vi "vi_tree.vi"   [LabVIEW 2010, in "zeromq.lvlib"]
uses:
  zeromq.lvlib
  poll_event_data.ctl
  zmq_context.lvclass
  zmq_socket.lvclass
  zmq_getsocketopt_int.vi
  zmq_poll_scalar.vi
panel:
  # "See back-panel for VI tree"
types:
  T1 = typedef "zeromq.lvlib/poll_event_data.ctl" = cluster{"identity":string, "data":string[]}
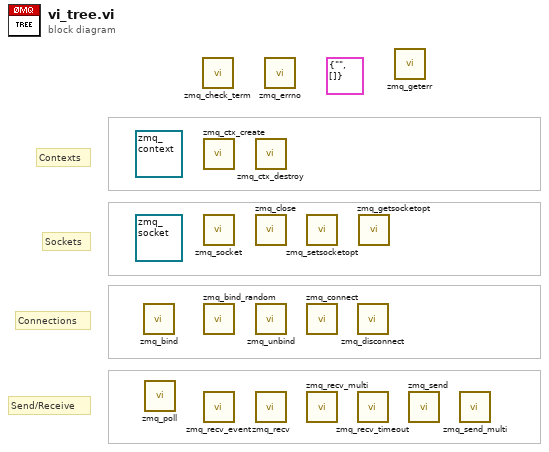
[diagram p0: block diagram]
diagram:
  (unwired) refnum<class "zmq_socket.lvclass"> refnum ("zeromq.lvlib:ZeroMQ Socket")
  (unwired) refnum<class "zmq_context.lvclass"> refnum ("zeromq.lvlib:ZeroMQ Context")
  (unwired) T1 {"identity"="", "data"=[]} ("poll data")
  # "Send/Receive"
  # "Connections"
  # "Sockets"
  # "Contexts"
  n1 = call "zmq_bind.vi"() -> ()  [unwired: 4 in, 2 out]
  n2 = call-poly "zmq_poll.vi"() -> ()  [unwired: 4 in, 4 out]
  n3 = call "zmq_check_term.vi"() -> ()  [unwired: 2 in, 2 out]
  n4 = call "zmq_ctx_create.vi"() -> ()  [unwired: 4 in, 2 out]
  n5 = call "zmq_socket.vi"() -> ()  [unwired: 5 in, 3 out]
  n6 = call "zmq_bind_random.vi"() -> ()  [unwired: 3 in, 3 out]
  n7 = call "zmq_recv_event.vi"() -> ()  [unwired: 6 in, 2 out]
  n8 = call "zmq_ctx_destroy.vi"() -> ()  [unwired: 5 in, 1 out]
  n9 = call "zmq_close.vi"() -> ()  [unwired: 5 in, 1 out]
  n10 = call "zmq_unbind.vi"() -> ()  [unwired: 4 in, 2 out]
  n11 = call "zmq_recv.vi"() -> ()  [unwired: 5 in, 5 out]
  n12 = call "zmq_errno.vi"() -> ()  [unwired: 2 in, 2 out]
  n13 = call "zmq_setsocketopt.vi"() -> ()  [unwired: 6 in, 2 out]
  n14 = call "zmq_connect.vi"() -> ()  [unwired: 4 in, 2 out]
  n15 = call "zmq_recv_multi.vi"() -> ()  [unwired: 3 in, 3 out]
  n16 = call "zmq_disconnect.vi"() -> ()  [unwired: 4 in, 2 out]
  n17 = call "zmq_recv_timeout.vi"() -> ()  [unwired: 4 in, 4 out]
  n18 = call-poly "zmq_getsocketopt.vi"() -> ()  [unwired: 3 in, 3 out]
  n19 = call "zmq_geterr.vi"() -> ()  [unwired: 1 in, 1 out]
  n20 = call "zmq_send.vi"() -> ()  [unwired: 7 in, 2 out]
  n21 = call "zmq_send_multi.vi"() -> ()  [unwired: 4 in, 2 out]
